vi "csv.vi"() -> ()   [LabVIEW 2016]
uses:
  <vilib>/Analysis/1siggen.llb/Ramp Pattern by Samples.vi
  <vilib>/Analysis/2dsp.llb/Real FFT.vi
  <vilib>/Utility/file.llb/Read From Spreadsheet File (string).vi
  <vilib>/gmath/NI_Gmath.lvlib
  <vilib>/Analysis/NI_AALBase.lvlib
  <vilib>/Analysis/NI_AALPro.lvlib
panel:
  out "PSD?":dbl[](graph)
  out "CHECK PEAK":cluster{i32[], dbl[]}[](graph)
  out "RRI":dbl[](graph)
  out "ORIGIN":cluster{dbl[], dbl[]}(graph)
  out "PEAK":cluster{i32[], dbl[]}(graph)
  out "Data Dsiplay 3":dbl[](array[numeric])
  out "Data Dsiplay 2":dbl[][](array[numeric])
  in  "CSV FILE PATH":path
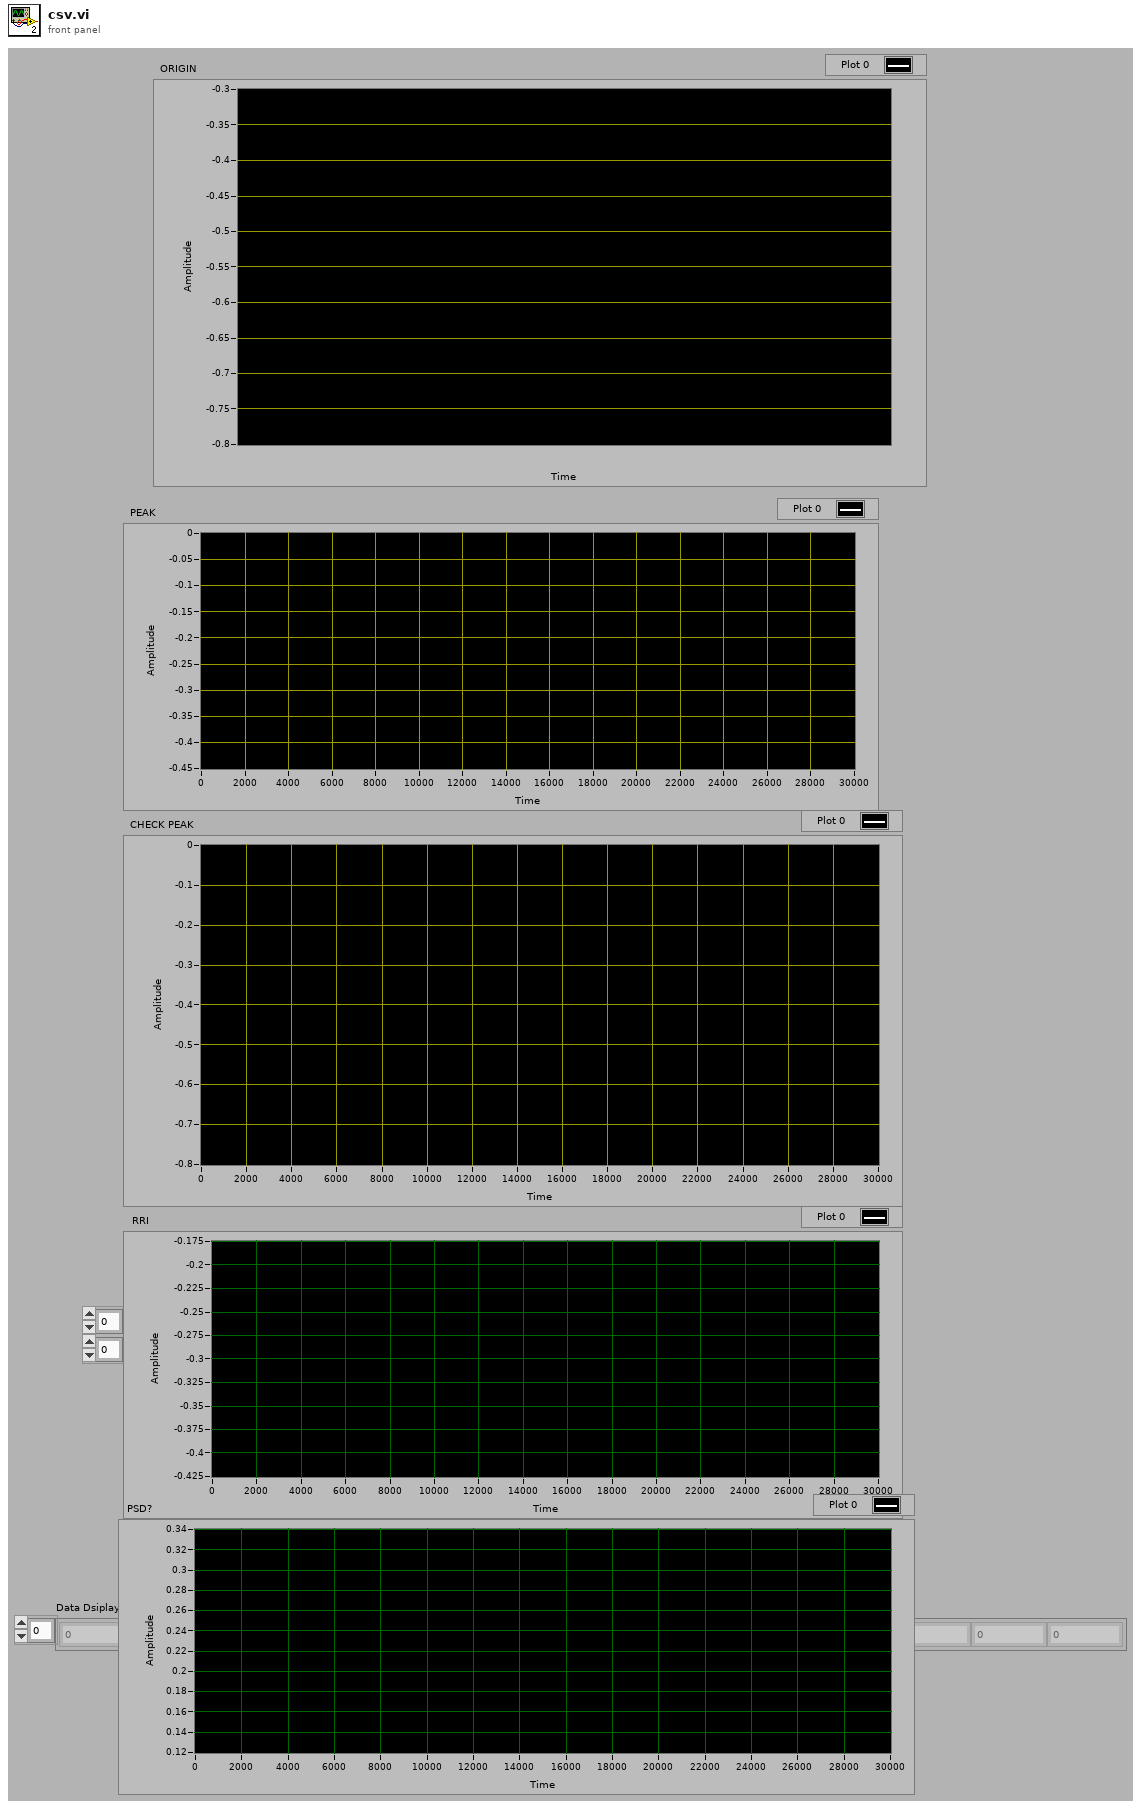
[diagram p1: front panel]
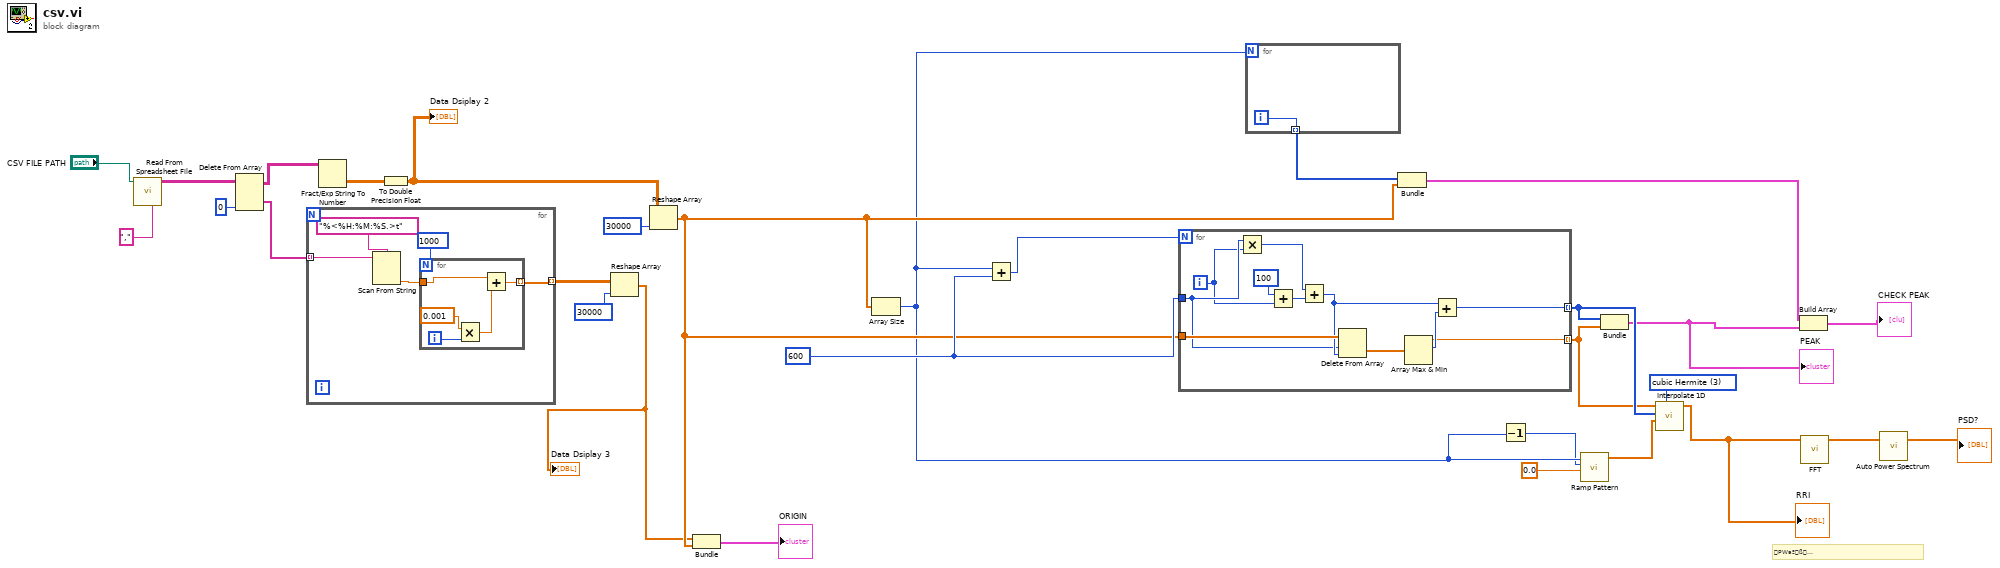
[diagram p0: block diagram]
diagram:
  w13 = 3 items=["nearest", "linear", "spline", "cubic Hermite", "Lagrange"] ("method")
  w19 = 600
  # "PWaºß\nNbvPEAKN#j"
  n1 = call-poly <vilib>:"Read From Spreadsheet File.vi"("delimiter (\\t)"="," ("delimiter (\\t)"), "file path (dialog if empty)"="CSV FILE PATH") -> ("all rows"=w28:string[][])  [unwired: 5 in, 4 out]
  n2 = Delete From Array(array=w28, index (col)=0 ("disabled index (col)")) -> (deleted portion=w24:string[], array with subset deleted=w25:string[][])  [unwired: 2 in]
  n3 = for {
    tunnel: w24 -> [w34] mode=indexing
    tunnel: [w31] -> w23 mode=indexing
    n4 = Scan From String(format string="%<%H:%M:%S.>t", input string=w34) -> (output 1=w33:dbl)  [unwired: 3 in, 3 out]
    n5 = for {
      N: 1000 -> [_]
      tunnel: w33 -> [w38]
      tunnel: [w36] -> w31 mode=indexing
      i -> [w39]
      n6 = Multiply(x=0.001, y=w39) -> (x*y=w37:dbl)
      n7 = Add(x=w38, y=w37) -> (x+y=w36:dbl)
    }
  }
  n8 = Fract/Exp String To Number(string=w25) -> (number=w26:dbl[][])  [unwired: 3 in, 1 out]
  n9 = To Double Precision Float(number=w26) -> (double precision float=w21:dbl[][])
  "Data Dsiplay 2" <- w21
  n10 = Reshape Array(w23, 30000 ("dimension size")) -> (w14:dbl[])
  "Data Dsiplay 3" <- w14
  n11 = Reshape Array(w21, 30000 ("dimension size")) -> (w15:dbl[])
  n12 = Bundle(w14, w15) -> (→"ORIGIN":cluster{dbl[], dbl[]})  [unwired: 1 in]
  n13 = Array Size(array=w15) -> (size(s)=w11:i32)
  n14 = Add(x=w11, y=w19) -> (x+y=w18:i32)
  n15 = for {
    N: w18 -> [_]
    tunnel: w15 -> [w51]
    tunnel: w19 -> [w45]
    tunnel: [w46] -> w12 mode=indexing
    tunnel: [w41] -> w4 mode=indexing
    i -> [w43]
    n16 = Multiply(x=w45, y=w43) -> (x*y=w42:i32)
    n17 = Add(x=100, y=w43) -> (x+y=w50:i32)
    n18 = Add(x=w42, y=w50) -> (x+y=w47:i32)
    n19 = Delete From Array(array=w51, length=w45, index=w47) -> (deleted portion=w49:dbl[])  [unwired: 1 out]
    n20 = Array Max & Min(array=w49) -> (max value=w41:dbl, max index (indices)=w48:i32)  [unwired: 2 out]
    n21 = Add(x=w47, y=w48) -> (x+y=w46:i32)
  }
  n22 = for {
    N: w11 -> [_]
    tunnel: [w52] -> w17 mode=indexing
    i -> [w52]
  }
  n23 = Bundle(w17, w15) -> (w7:cluster{i32[], dbl[]})  [unwired: 1 in]
  n24 = Decrement(x=w11) -> (x-1=w10:i32)
  n25 = call-poly <vilib>:"Ramp Pattern.vi"("start"=0.0, "end"=w10, "samples"=w11) -> ("Ramp Pattern"=w8:dbl[])  [unwired: 7 in, 1 out]
  n26 = Bundle(w12, w4) -> (w6:cluster{i32[], dbl[]})  [unwired: 1 in]
  "PEAK" <- w6
  n27 = call <vilib>:"Interpolate 1D.vi"("method"=w13, "xi"=w8, "X"=w12, "Y"=w4) -> ("yi"=w3:dbl[])  [unwired: 5 in, 2 out]
  "RRI" <- w3
  n28 = Build Array "Build Array"(w7, w6) -> (→"CHECK PEAK":cluster{i32[], dbl[]}[])
  n29 = call-poly <vilib>:"FFT.vi"("X"=w3) -> ("FFT {X}"=w2:cdb[])  [unwired: 9 in, 1 out]
  n30 = call <vilib>:"Auto Power Spectrum.vi"("Signal (V)"=w2) -> ("Power Spectrum (V^2 rms)"=→"PSD?":dbl[])  [unwired: 1 in, 1 out]
